vi "update std eng cluster.vi"(11 "Engine Configuration in":T9) -> (3 "Engine Configuration out":T1={"Loop Info"={"Processor"=0, "Priority"=0, "timing source type"=enum."1 MHz Clock", "module providing source"="", "timing source dt"=5000, "timing policy"=enum."nonblocking"}, "Module Specific Configuration"=[]})   [LabVIEW 2013, in "Standard Engine Configuration.lvclass"]
uses:
  Standard Engine Configuration.lvclass
  Engine Configuration.ctl
  Loop Info.ctl
  Supported Timing Sources.ctl
  timing policy.ctl
  Module Specific Configuration.ctl
  Module Decimation.ctl
  Runtime/error responses.ctl
  error options.ctl
  <vilib>/NI/DCAF Module Framework/runtime/error classification.ctl
  Error Actions.ctl
  <vilib>/NI/DCAF Module Framework/runtime/TBM module execution interface.lvclass
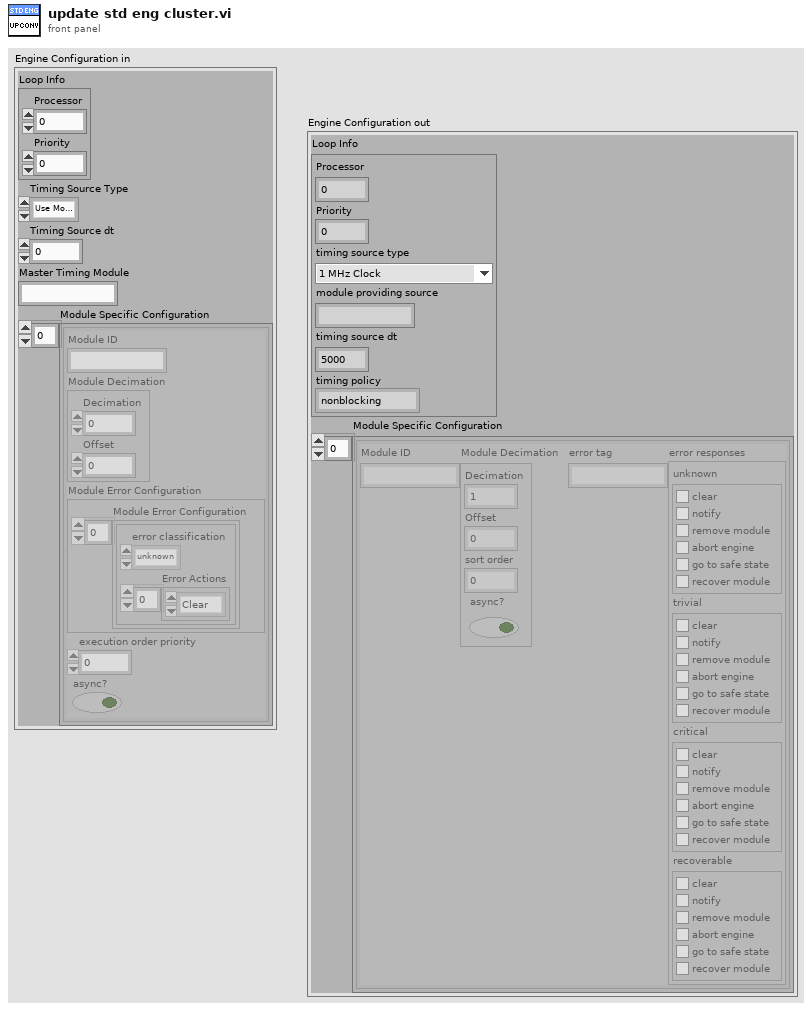
[diagram p1: front panel]
types:
  T1 = typedef "Standard Engine Configuration.lvclass/Engine Configuration.ctl" = cluster{"Loop Info":T2, "Module Specific Configuration":T5[]}
  T2 = typedef "Standard Engine Configuration.lvclass/Loop Info.ctl" = cluster{"Processor":i32, "Priority":i32, "timing source type":T3, "module providing source":string, "timing source dt":u32, "timing policy":T4}
  T3 = typedef "Standard Engine Configuration.lvclass/Supported Timing Sources.ctl" = enum16{"Use Module Timing Source", "1 kHz Clock", "1 MHz Clock", "Synchronize to Scan Engine"}
  T4 = typedef "Standard Engine Configuration.lvclass/timing policy.ctl" = enum16{"strict determinism", "nonblocking", "nondeterministic inline"}
  T5 = typedef "Standard Engine Configuration.lvclass/Module Specific Configuration.ctl" = cluster{"Module ID":string, "Module Decimation":T6, "error tag":string, "error responses":T7}
  T6 = typedef "Standard Engine Configuration.lvclass/Module Decimation.ctl" = cluster{"Decimation":u16, "Offset":u16, "sort order":i32, "async?":bool}
  T7 = typedef "Standard Engine Configuration.lvclass/error responses.ctl" = cluster{"unknown":T8, "trivial":T8, "critical":T8, "recoverable":T8}
  T8 = typedef "Standard Engine Configuration.lvclass/error options.ctl" = cluster{"clear":bool, "notify":bool, "remove module":bool, "abort engine":bool, "go to safe state":bool, "recover module":bool}
  T9 = cluster{"Loop Info":cluster{"Processor":i32, "Priority":i32}, "Timing Source Type":enum16{"Use Module Timing Source", "1 kHz Clock", "1 MHz Clock", "Synchronize to Scan Engine"}, "Timing Source dt":u32, "Master Timing Module":string, "Module Specific Configuration":cluster{"Module ID":string, "Module Decimation":cluster{"Decimation":u16, "Offset":u16}, "Module Error Configuration":cluster{"Module Error Configuration":cluster{"error classification":enum16{"unknown", "none", "trivial", "recoverable", "critical"}, "Error Actions":enum16{"Clear", "Notify", "Stop Component", "Stop Engine", "Safe State", "Attempt Recovery"}[]}[]}, "execution order priority":i32, "async?":bool}[]}
  T10 = typedef "TBM module execution interface.lvclass/error classification.ctl" = enum16{"unknown", "none", "trivial", "recoverable", "critical"}
  T11 = typedef "Standard Engine Configuration.lvclass/Error Actions.ctl" = enum16{"Clear", "Notify", "Stop Component", "Stop Engine", "Safe State", "Attempt Recovery"}
  T12 = cluster{"Loop Info":cluster{"Processor":i32, "Priority":i32}, "Timing Source Type":T3, "Timing Source dt":u32, "Master Timing Module":string, "Module Specific Configuration":cluster{"Module ID":string, "Module Decimation":cluster{"Decimation":u16, "Offset":u16}, "Module Error Configuration":cluster{"Module Error Configuration":cluster{"error classification":T10, "Error Actions":T11[]}[]}, "execution order priority":i32, "async?":bool, "error tag":string}[]}
  T13 = enum16{"Use Module Timing Source", "1 kHz Clock", "1 MHz Clock", "Synchronize to Scan Engine"}
  T14 = cluster{"Module ID":string, "Module Decimation":cluster{"Decimation":u16, "Offset":u16}, "Module Error Configuration":cluster{"Module Error Configuration":cluster{"error classification":enum16{"unknown", "none", "trivial", "recoverable", "critical"}, "Error Actions":enum16{"Clear", "Notify", "Stop Component", "Stop Engine", "Safe State", "Attempt Recovery"}[]}[]}, "execution order priority":i32, "async?":bool}[]
  T15 = cluster{"Module ID":string, "Module Decimation":cluster{"Decimation":u16, "Offset":u16}, "Module Error Configuration":cluster{"Module Error Configuration":cluster{"error classification":T10, "Error Actions":T11[]}[]}, "execution order priority":i32, "async?":bool, "error tag":string}
  T16 = cluster{"Module Error Configuration":cluster{"error classification":enum16{"unknown", "none", "trivial", "recoverable", "critical"}, "Error Actions":enum16{"Clear", "Notify", "Stop Component", "Stop Engine", "Safe State", "Attempt Recovery"}[]}[]}
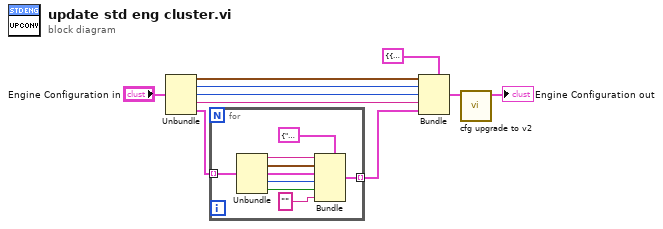
[diagram p0: block diagram]
diagram:
  n1 = Unbundle("Engine Configuration in") -> ("Loop Info"=w7:cluster{"Processor":i32, "Priority":i32}, "Timing Source Type"=w6:T13, "Timing Source dt"=w5:u32, "Master Timing Module"=w4:string, "Module Specific Configuration"=w9:T14)
  n2 = for {
    tunnel: w9 -> [w19] mode=indexing
    tunnel: [w18] -> w8 mode=indexing
    n3 = Unbundle(w19) -> ("Module ID"=w17:string, "Module Decimation"=w16:cluster{"Decimation":u16, "Offset":u16}, "Module Error Configuration"=w15:T16, "execution order priority"=w14:i32, "async?"=w13:bool)
    n4 = Bundle(cluster=T15 {"Module ID"="", "Module Decimation"={"Decimation"=1, "Offset"=0}, "Module Error Configuration"={"Module Error Configuration"=[]}, "execution order priority"=0, "async?"=FALSE, "error tag"=""} ("Module Specific Configuration"), "Module ID"=w17, "Module Decimation"=w16, "Module Error Configuration"=w15, "execution order priority"=w14, "async?"=w13, "error tag"="") -> (w18:T15)
  }
  n5 = Bundle(cluster=T12 {"Loop Info"={"Processor"=-2, "Priority"=1}, "Timing Source Type"=enum."1 kHz Clock", "Timing Source dt"=5, "Master Timing Module"="", "Module Specific Configuration"=[]} ("Engine Configuration"), "Loop Info"=w7, "Timing Source Type"=w6, "Timing Source dt"=w5, "Master Timing Module"=w4, "Module Specific Configuration"=w8) -> (w1:T12)
  n6 = call "cfg upgrade to v2.vi"("Engine Configuration"=w1) -> ("Engine Configuration out"=→"Engine Configuration out":T1)  [unwired: 10 in]
